vi "2D_String_array_from_string.vi"(1 "String Name":string, 2 "Input string":string, 3 "Array title":string) -> (0 "2D data array":string[][](array[string]))   [LabVIEW 2010]
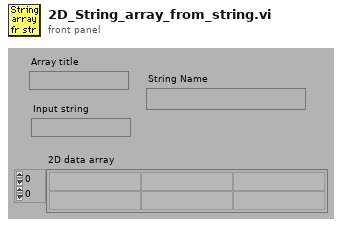
[diagram p1: front panel]
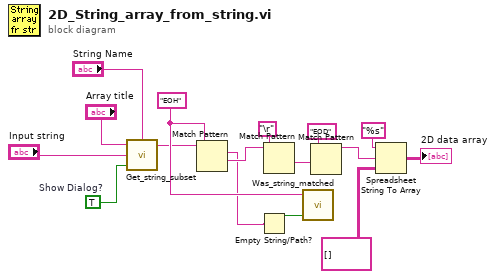
[diagram p0: block diagram]
diagram:
  w2 = TRUE  # Show Dialog?
  w9 = "EOH"
  n1 = call "Get_string_subset.vi"("String Name"="String Name", "Show Dialog?"=w2, "String to split"="Input string", "File Label"="Array title") -> ("Output string"=w8:string)  [unwired: 1 out]
  n2 = Match Pattern(string=w8, regular expression=w9) -> (match substring=w4:string, after substring=w16:string)  [unwired: 3 out]
  n3 = Empty String/Path?(string/path=w4) -> (empty?=w3:bool)
  n4 = Match Pattern(string=w16, regular expression="\r") -> (after substring=w15:string)  [unwired: 4 out]
  n5 = call "Was_string_matched.vi"("Match Error"=w3, "Variable name"=w9) -> ()  [unwired: 1 in]
  n6 = Match Pattern(string=w15, regular expression="EOD") -> (before substring=w13:string)  [unwired: 4 out]
  n7 = Spreadsheet String To Array(format string="%s", spreadsheet string=w13, array type (2D Dbl)=string[][] []) -> (array=→"2D data array":string[][])  [unwired: 1 out]
